vi "configureVDCRange.vi"(0 "NInstrSim":refnum<class "NInstrSim.lvclass">, 2 "DC Voltage Range (1:10 VDC)":u16(ring)=1 items=["0:1 VDC", "0:10 VDC", "0:100 VDC"], 5 "error in (no error)":errorcluster) -> (14 "dup NInstrSim":refnum<class "NInstrSim.lvclass">, 19 "error out":errorcluster)   [LabVIEW 2009, in "HB_Device_Examples.lvlib" / "NInstrSim.lvclass"]
doc: "Configures the range of DC Voltage values generated by the NI Instrument Simulator."
uses:
  NInstrSim.lvclass
  lib.lib/HGF_LVC/HGF_DeviceBaseClasses/HGF_VISADevice/HGF_VISADevice.lvclass
  non_GPL/instr.lib/NI Instrument Simulator/NI Instrument Simulator.lvlib
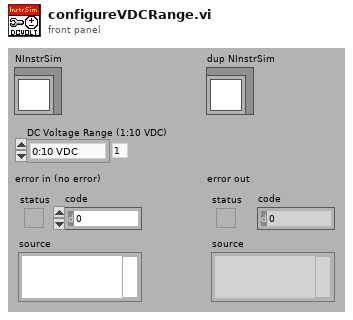
[diagram p1: front panel]
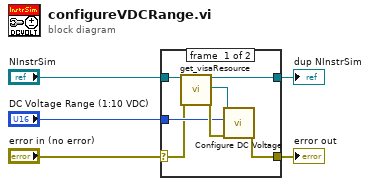
[diagram p0: block diagram]
diagram:
  n1 = case shown="No Error" "error in (no error)" {
    selector: "error in (no error)" -> [w7 w14]
    tunnel: [w6 w14] -> w4
    tunnel: [w11 w13] -> w2
    tunnel: "NInstrSim" -> [w12 w13]
    tunnel: "DC Voltage Range (1:10 VDC)" -> [w8 _]
    frame #0 {
      n2 = call "get_visaResource.vi"("HGF_VISADevice"=w12, "error in (no error)"=w7) -> ("dup HGF_VISADevice"=w11:refnum<class "NInstrSim.lvclass">, "VISA Resource Name"=w10:refnum<visa-resource-name>, "error out"=w9:errorcluster)  [unwired: 15 out]
      n3 = call "Configure DC Voltage.vi"("error in (no error)"=w9, "DC Voltage Range (1:10 VDC)"=w8, "VISA resource name"=w10) -> ("error out"=w6:errorcluster)  [unwired: 8 out]
    }
    frame #1 {
    }
  }
  "error out" <- w4
  "dup NInstrSim" <- w2
